vi "Init RemoteDataService.vi"(8 "error in (no error)":errorcluster, 11 "Vecto in":refnum<class "Vecto.lvclass">) -> (0 "error out":errorcluster, 3 "Vecto out":refnum<class "Vecto.lvclass">)   [LabVIEW 2020, in "Vecto.lvlib" / "Vecto.lvclass"]
uses:
  Vecto.lvclass
  Vecto.lvclass/Vecto.ctl
  RemoteDataService/RemoteDataService.lvclass
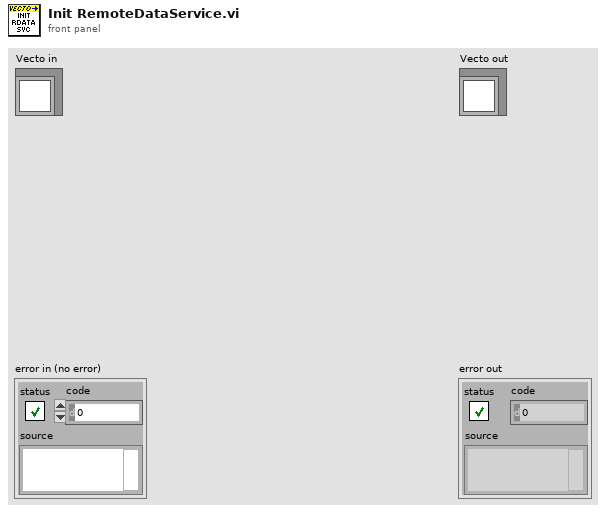
[diagram p1: front panel]
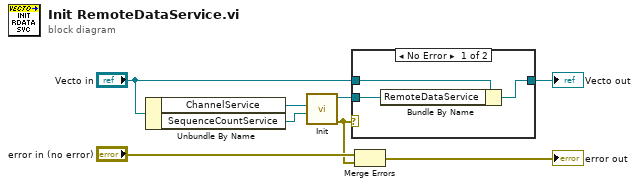
[diagram p0: block diagram]
diagram:
  n1 = Unbundle By Name("Vecto in") -> ("ChannelService"=w3:refnum<class "ChannelService.lvclass">, "SequenceCountService"=w2:refnum<class "SequenceCountService.lvclass">)
  n2 = call "Init.vi"("SequenceCountService"=w2, "ChannelService"=w3) -> ("error out"=w1:errorcluster, "RemoteDataService out"=w5:refnum<class "RemoteDataService.lvclass">)  [unwired: 8 in]
  n3 = case shown="No Error" w1 {
    tunnel: w5 -> [w11 _]
    tunnel: "Vecto in" -> [w9 w12]
    tunnel: [w10 w12] -> w7
    frame No Error {
      n4 = Bundle By Name(cluster=w9, "RemoteDataService"=w11) -> (w10:refnum<class "Vecto.lvclass">)
    }
    frame Error {
    }
  }
  "Vecto out" <- w7
  n5 = Merge Errors("error in (no error)", w1) -> (→"error out":errorcluster)
